vi "UnscentedKalmanFilter_New_Default.vi"(4 "Inputs":i32, 5 "States":i32, 6 "dt_Seconds":dbl=0.02, 7 "Outputs":i32, 10 "MeasurementStdDevs":T1, 11 "StateStdDevs":T1) -> (0 "Error":errorcluster, 3 "UnscentedKalmanFiilter":T2)   [LabVIEW 2019, in "Trajectory_Library.lvlib"]
doc: "A Kalman filter combines predictions from a model and measurements to give an estimate of the true ystem state. This is useful because many states cannot be measured directly as a result of sensor noise, or because the state is \"hidden\".\n \nThe Unscented Kalman filter is similar to the Kalman filter, except that it propagates carefully chosen points called sigma points through the non-linear model to obtain an estimate of the true covariance (as opposed to a linearized version of it). This means that the UKF works with nonlinear systems.\n \nConstructs an unscented Kalman filter with custom mean, residual, and addition functions. Using custom functions for arithmetic can be useful if you have angles in the state or measurements, because they allow you to correctly account for the modular nature of angle arithmetic.\n\nConstructs an Unscented Kalman Filter.\n \nInputs:\n - states -- The number of states.\n - outputs -- The number of outputs.\n - stateStdDevs -- Standard deviations of model states.\n - measurementStdDevs -- Standard deviations of measurements.\n - nominalDtSeconds -- Nominal discretization timestep.\n - Inputs -- the number of inputs.\n\nOutputs:\n - outUnscentedKalmanFilter -- updated filter data cluster\n - Error -- If TRUE, an error occured."
uses:
  Trajectory_Library.lvlib
  UNSCENTED_KALMAN_FILTER.ctl
  <vilib>/Analysis/Matrix/Datatypes/RealMatrix.ctl
  MERWE_SCALED_SIGMA_PTS.ctl
  CALLBACK_FUNC_TYPE.ctl
  <vilib>/Analysis/Matrix/NI_Matrix.lvlib
panel:
  # "<States,1>"
  # "<Outputs,1>"
  # "State Estimate <Statess,1>"
  # "<States, States>"
  # "<States, ?>"
  # "<Statess,  States>"
  # "<Outputs, Outputs>"
  # "<?, 1>"
  # "<?, 1>"
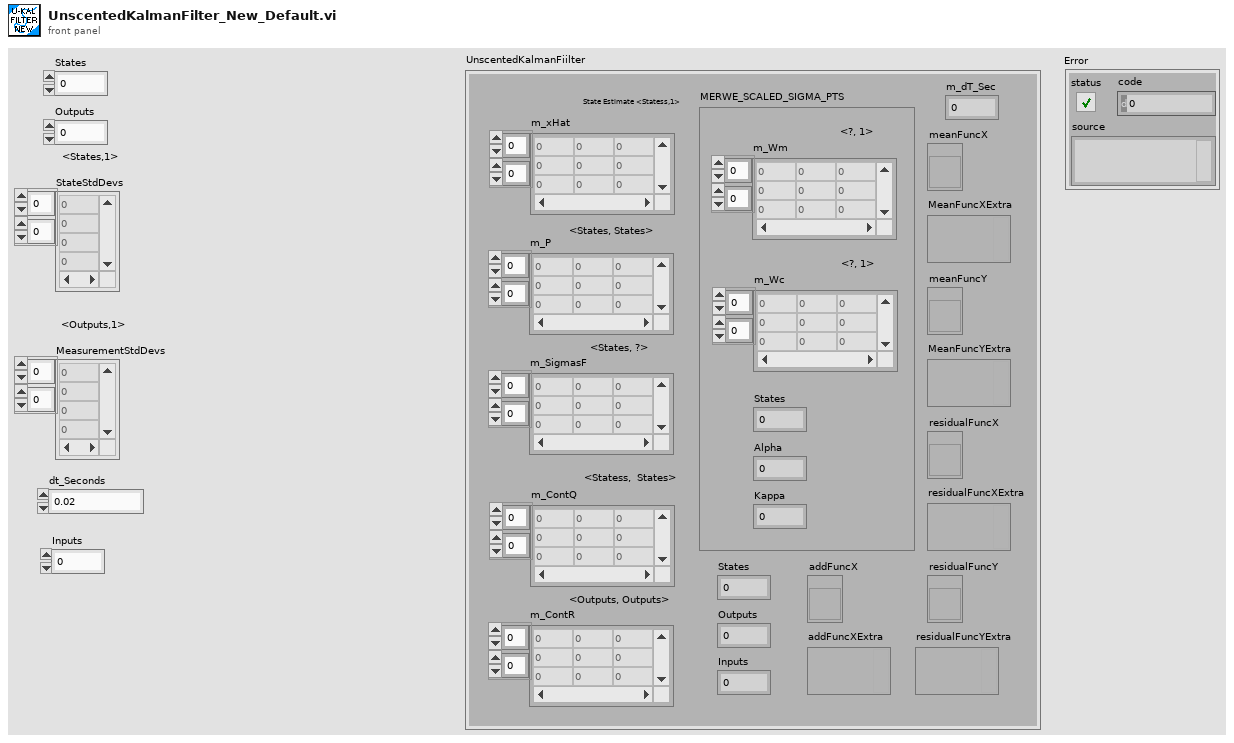
[diagram p1: front panel]
types:
  T1 = typedef "NI_Matrix.lvlib/RealMatrix.ctl" = dbl[][]
  T2 = typedef "Trajectory_Library.lvlib/UNSCENTED_KALMAN_FILTER.ctl" = cluster{"m_P":T1, "m_xHat":T1, "States":i32, "Outputs":i32, "m_ContR":T1, "m_ContQ":T1, "m_SigmasF":T1, "m_dT_Sec":dbl, "MERWE_SCALED_SIGMA_PTS":T3, "meanFuncX":T4, "meanFuncY":T4, "residualFuncX":T4, "residualFuncY":T4, "addFuncX":T4, "addFuncXExtra":variant, "residualFuncYExtra":variant, "residualFuncXExtra":variant, "MeanFuncYExtra":variant, "MeanFuncXExtra":variant, "Inputs":i32}
  T3 = typedef "Trajectory_Library.lvlib/MERWE_SCALED_SIGMA_PTS.ctl" = cluster{"m_Wm":T1, "States":i32, "Alpha":dbl, "m_Wc":T1, "Kappa":i32}
  T4 = typedef "Trajectory_Library.lvlib/CALLBACK_FUNC_TYPE.ctl" = refnum<vi>
  T5 = typedef "Trajectory_Library.lvlib/UNSCENTED_KALMAN_NEW_FUNC_GROUP.ctl" = cluster{"meanFuncX":T4, "meanFuncY":T4, "residualFuncX":T4, "residualFuncY":T4, "addFuncX":T4, "MeanFuncXExtra":variant, "MeanFuncYExtra":variant, "residualFuncXExtra":variant, "residualFuncYExtra":variant, "addFuncXExtra":variant}
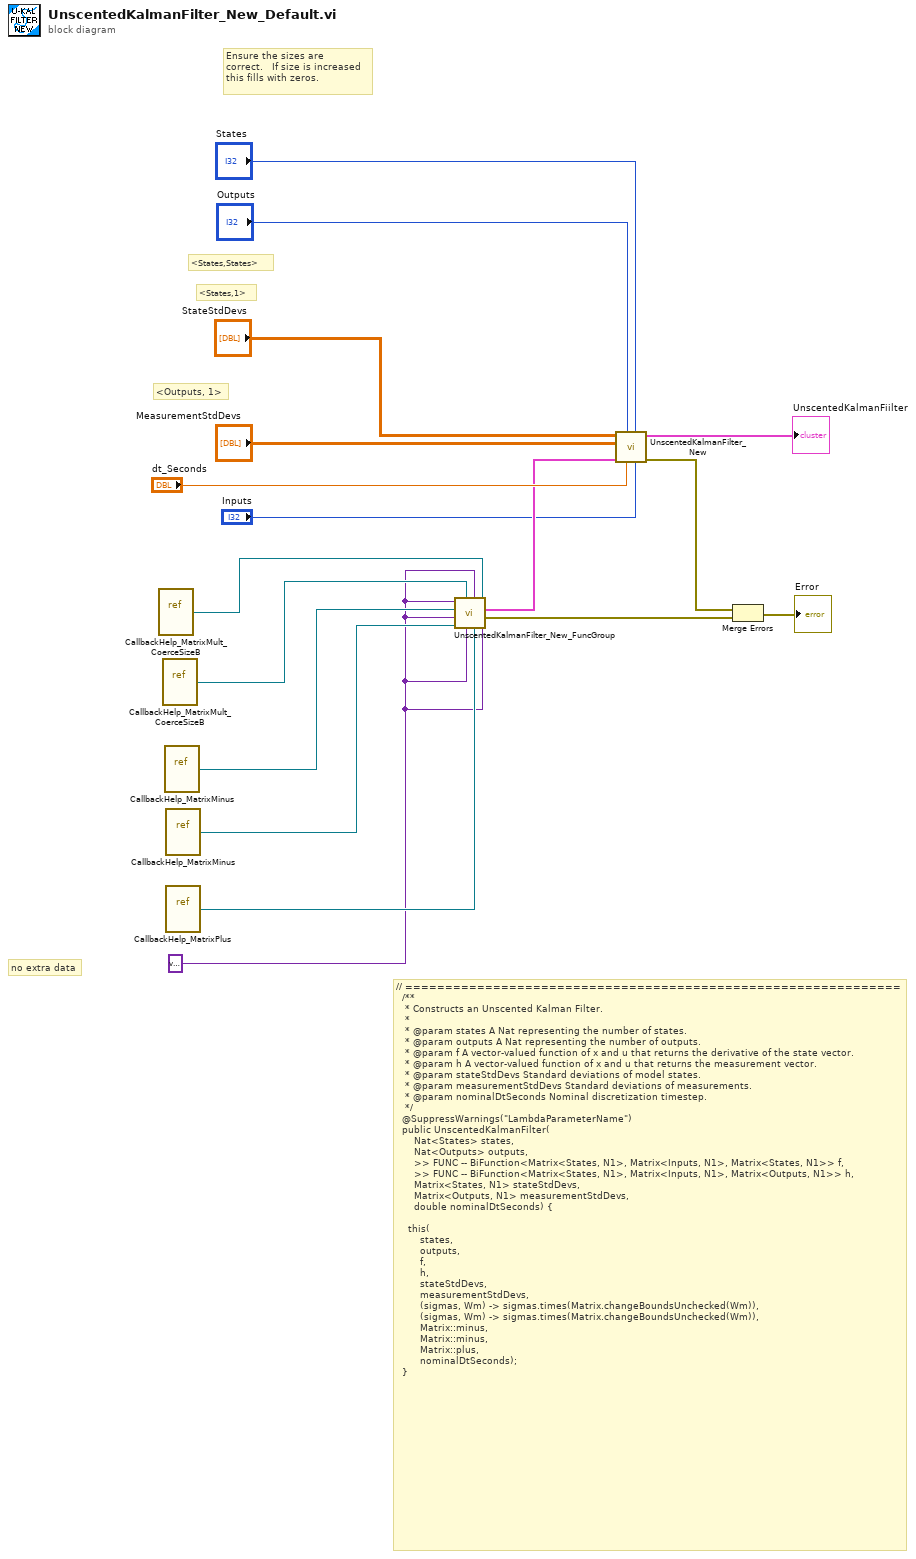
[diagram p0: block diagram]
diagram:
  w2 = variant ("addFuncXExtra")
  # "no extra data"
  # "// ==============================================================\n  /**\n   * Constructs an Unscented Kalman Filter.\n   *\n   * @param states A Nat representing the number of states.\n   * @param outputs A Nat representing the number of outputs.\n   * @param f A vector-valued function of x and u that returns the derivative of the state vector.\n   * @param h A vector-valued function of x and u that returns the measurement vector.\n   * @param stateStdDevs Standard deviations of model states.\n   * @param measurementStdDevs Standard deviations of measurements.\n   * @param nominalDtSeconds Nominal discretization timestep.\n   */\n  @SuppressWarnings(\"LambdaParameterName\")\n  public UnscentedKalmanFilter(\n      Nat<States> states,\n      Nat<Outputs> outputs,\n      >> FUNC -- BiFunction<Matrix<States, N1>, Matrix<Inputs, N1>, Matrix<States, N1>> f,\n      >> FUNC -- BiFunction<Matrix<States, N1>, Matrix<Inputs, N1>, Matrix<Outputs, N1>> h,\n      Matrix<States, N1> stateStdDevs,\n      Matrix<Outputs, N1> measurementStdDevs,\n      double nominalDtSeconds) {\n\n    this(\n        states,\n        outputs,\n        f,\n        h,\n        stateStdDevs,\n        measurementStdDevs,\n        (sigmas, Wm) -> sigmas.times(Matrix.changeBoundsUnchecked(Wm)),\n        (sigmas, Wm) -> sigmas.times(Matrix.changeBoundsUnchecked(Wm)),\n        Matrix::minus,\n        Matrix::minus,\n        Matrix::plus,\n        nominalDtSeconds);\n  }"
  # "<Outputs, 1>"
  # "<States,1>"
  # "<States,States>"
  # "Ensure the sizes are\ncorrect.   If size is increased \nthis fills with zeros."
  n1 = vi-ref "CallbackHelp_MatrixMult_CoerceSizeB.vi"() -> (w3:refnum<vi>)
  n2 = vi-ref "CallbackHelp_MatrixMult_CoerceSizeB.vi"() -> (w4:refnum<vi>)
  n3 = vi-ref "CallbackHelp_MatrixMinus.vi"() -> (w6:refnum<vi>)
  n4 = vi-ref "CallbackHelp_MatrixMinus.vi"() -> (w5:refnum<vi>)
  n5 = vi-ref "CallbackHelp_MatrixPlus.vi"() -> (w7:refnum<vi>)
  n6 = call "UnscentedKalmanFilter_New_FuncGroup.vi"("addFuncXExtra"=w2, "MeanFuncX"=w3, "AddFuncX"=w7, "MeanFuncXExtra"=w2, "residualFuncYExtra"=w2, "MeanFuncY"=w4, "ResidualFuncY"=w5, "residualFuncXExtra"=w2, "ResidualFuncX"=w6, "MeanFuncYExtra"=w2) -> ("Error"=w14:errorcluster, "UNSCENTED_KALMAN_NEW_FUNC_GROUP"=w8:T5)
  n7 = call "UnscentedKalmanFilter_New.vi"("Inputs"="Inputs", "States"="States", "dt_Seconds"="dt_Seconds", "Outputs"="Outputs", "UNSCENTED_KALMAN_NEW_FUNC_GROUP"=w8, "MeasurementStdDevs"="MeasurementStdDevs", "StateStdDevs"="StateStdDevs") -> ("Error"=w16:errorcluster, "UnscentedKalmanFiilter"=→"UnscentedKalmanFiilter":T2)  [unwired: 3 in]
  n8 = Merge Errors(w16, w14) -> (→"Error":errorcluster)
